vi "chooseStates.vi"(7 "First call?":bool, 9 "Robot":refnum<class "Robot.lvclass">, 10 "Game in":refnum<class "Game.lvclass">, 11 "ReceivePassInFuturePointTactic in":refnum<class "ReceivePassInFuturePointTactic.lvclass">) -> (0 "FuturePointToGo":dbl[](array[numeric]), 1 "StateToExecute":enum16{"Exit", "Halt", "GoTo"}(ring), 2 "ExitTactic?":bool, 3 "ReceivePassInFuturePointTactic out":refnum<class "ReceivePassInFuturePointTactic.lvclass">)   [LabVIEW 2020, in "ReceivePassInFuturePointTactic.lvclass"]
uses:
  ReceivePassInFuturePointTactic.lvclass
  KickToPassReceiverTactic_class/KickToPassReceiverTactic.lvclass
  Utilities_class/Utilities.lvclass
  Robot_class/roles.ctl
  Game_class/Game.lvclass
  Robot_class/Robot.lvclass
  Ball_class/Ball.lvclass
  Ally_class/Ally.lvclass
  Parameters_class/Parameters.lvclass
  Field_class/Field.lvclass
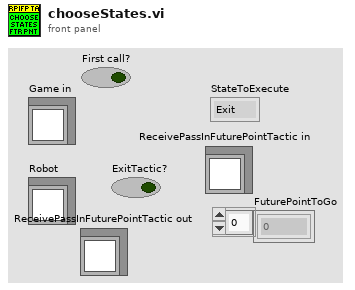
[diagram p1: front panel]
types:
  T1 = typedef "roles.ctl" = enum16{"SecondMarker", "WaitPass", "ABCThirdKicker", "ABCFirstKicker", "ABCSecondKicker", "Tabler", "TableFinalizer", "PrepareRollToPassRoller", "PrepareRollToPassReceiver", "SimplePassRoll", "SimplePassRollReceiver", "PenaltyDefense", "PreparePassReceiver 2", "PreparePassReceiver 1", "PassObserver", "Timeout", "Goto", "ZigZag", "None", "BallOutOfField", "DefenderArea", "Duelist", "AttackerStop", "FollowAttacker", "KeeperRole", "KickPenalty", "AttackerAimGoal", "AttackerBlock", "Marker", "Halt", "Shoot", "PassKicker", "PassReceiver", "TestRole", "PenaltyAttacker"}
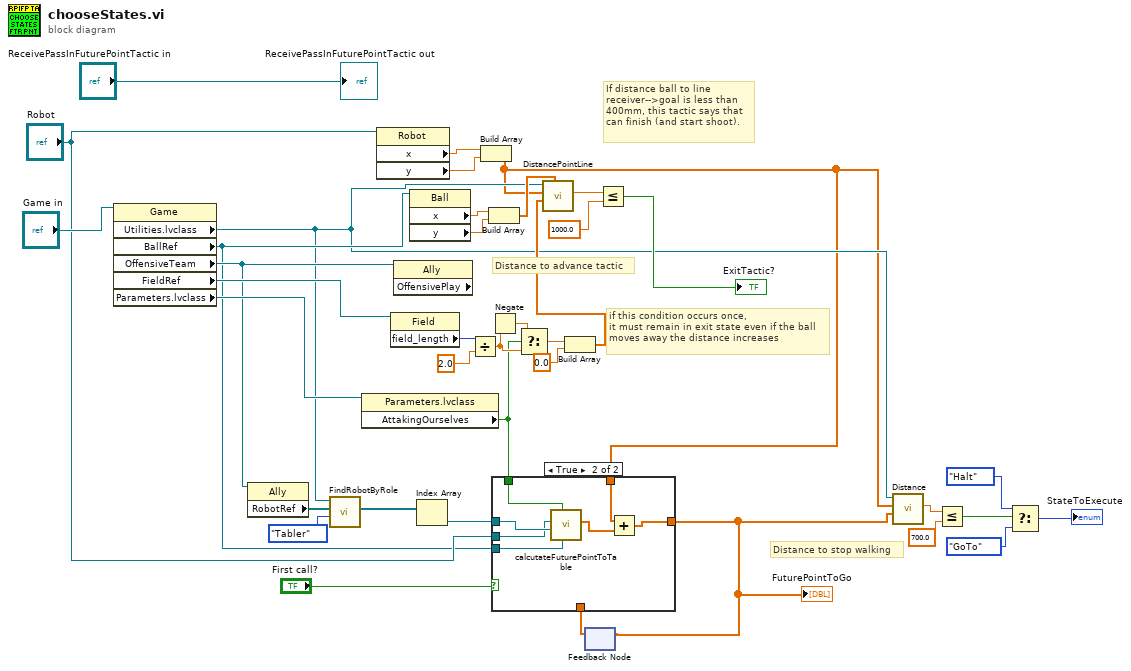
[diagram p0: block diagram]
diagram:
  # "Distance to stop walking"
  # "Distance to advance tactic"
  # "if this condition occurs once,\nit must remain in exit state even if the ball\nmoves away the distance increases"
  # "If distance ball to line\nreceiver-->goal is less than\n400mm, this tactic says that\ncan finish (and start shoot)."
  n1 = property class="Game"(reference="Game in") -> ("Utilities.lvclass"=w10:refnum<class "Utilities.lvclass">, "BallRef"=w13:refnum<class "Ball.lvclass">, "OffensiveTeam"=w16:refnum<class "Ally.lvclass">, "FieldRef"=w30:refnum<class "Field.lvclass">, "Parameters.lvclass"=w33:refnum<class "Parameters.lvclass">)  [unwired: 1 in, 2 out]
  n2 = property class="Ally"(reference=w16) -> ("RobotRef"=w15:refnum<class "Robot.lvclass">[])  [unwired: 1 in, 2 out]
  n3 = call "FindRobotByRole.vi"("role"=roles."Tabler", "RobotRef"=w15, "Utilities in"=w10) -> ("Robots"=w19:refnum<class "Robot.lvclass">[])  [unwired: 6 in, 2 out]
  n4 = property class="Parameters.lvclass"(reference=w33) -> ("AttakingOurselves"=w20:bool)  [unwired: 1 in, 2 out]
  n5 = property class="Robot"(reference="Robot") -> ("x"=w24:dbl, "y"=w25:dbl)  [unwired: 1 in, 2 out]
  n6 = property class="Field"(reference=w30) -> ("field_length"=w31:i32)  [unwired: 1 in, 2 out]
  n7 = property class="Ally" props=["OffensivePlay"](reference=w16) -> ()  [unwired: 1 in, 3 out]
  n8 = property class="Ball"(reference=w13) -> ("x"=w22:dbl, "y"=w23:dbl)  [unwired: 1 in, 2 out]
  n9 = Index Array(array=w19) -> (element=w18:refnum<class "Robot.lvclass">)  [unwired: 1 in]
  n10 = Divide(x=w31, y=2.0) -> (x/y=w35:dbl)
  n11 = Build Array(w24, w25) -> (w2:dbl[])
  n12 = Build Array(w22, w23) -> (w29:dbl[])
  n13 = Negate(x=w35) -> (-x=w34:dbl)
  n14 = Select(t=w34, s=w20, f=w35) -> (s? t:f=w36:dbl)
  n15 = Build Array(w36, 0.0) -> (w38:dbl[])
  n16 = call-dynamic "DistancePointLine.vi"("Q"=w29, "P2"=w38, "P1"=w2, "Utilities in"=w10) -> ("distance"=w26:dbl)  [unwired: 5 in, 2 out]
  n17 = feedback #1() -> (w12:dbl[])  [unwired: 1 in]
  n18 = case shown="True" "First call?" {
    tunnel: w20 -> [_ w46]
    tunnel: w18 -> [_ w44]
    tunnel: "Robot" -> [_ w43]
    tunnel: w13 -> [_ w45]
    tunnel: [w39 w40] -> w1
    tunnel: w12 -> [w39 _]
    tunnel: w2 -> [_ w41]
    frame False {
    }
    frame True {
      n19 = call "calcutateFuturePointToTable.vi"("BallRef"=w45, "AttackingOurselves?"=w46, "Robot that\nmake the pass"=w44, "Robot that will\nreceive the pass"=w43) -> ("Array to Receiver trajectory"=w42:dbl[])  [unwired: 5 in, 2 out]
      n20 = Add(x=w41, y=w42) -> (x+y=w40:dbl[])
    }
  }
  "FuturePointToGo" <- w1
  n21 = feedback-in #1(w1) -> ()
  n22 = Less Or Equal?(x=w26, y=1000.0) -> (x <= y?=→"ExitTactic?":bool)
  n23 = call-dynamic "Distance.vi"("P1"=w1, "P2"=w2, "Utilities in"=w10) -> ("Distance"=w9:dbl)  [unwired: 6 in, 2 out]
  n24 = Less Or Equal?(x=w9, y=700.0) -> (x <= y?=w7:bool)
  n25 = Select(t=enum16{"Exit", "Halt", "GoTo"}."Halt" ("States"), s=w7, f=enum16{"Exit", "Halt", "GoTo"}."GoTo" ("States")) -> (s? t:f=→"StateToExecute":enum16{"Exit", "Halt", "GoTo"})
  "ReceivePassInFuturePointTactic out" <- "ReceivePassInFuturePointTactic in"
